vi "Read From I16 File.vi"(8 "start of read offset (bytes:0)":i32 caption="Start des Lese-Offset (Byte:0)", 9 "2D number of columns/1D count (all as 1D:-1)":i32=-1 caption="2D Spaltenanzahl/1D Anzahl (alle als 1D:-1)", 10 "2D number of rows":i32 caption="2D-Zeilenanzahl", 11 "file path (dialog if empty)":path caption="Dateipfad (Dialog, wenn leer)") -> (0 "mark after read (bytes)":i32 caption="Dateimarke nach Lesevorgang (Byte)", 1 "1D array":i16[](array[numeric]) caption="1D-Array", 2 "2D array":i16[][](array[numeric]) caption="2D-Array", 3 "new file path (Not A Path if cancelled)":path caption="Neuer Dateipfad (Kein Pfad, wenn abgebrochen)", 4 "EOF?":bool caption="Dateiende?")   [LabVIEW 2009]
doc: "Liest ein 2D- oder 1D-Daten-Array aus einer Bytestream-Datei mit vorzeichenbehafteten Word-Integern (I16) aus."
panel:
  in  "prompt":string="Zu lesende Datei wählen." caption="Eingabeaufforderung"
  in  "instructions":string="* Um die ganze Datei in ein 1D Array einzulesen, den 1D Zähler auf <0 (Standard) stellen ; Sie können die 2D Zeilenanzahl unverdrahtet lassen.\n* Zum Einlesen von N-Elementen in ein 1D Array, den 1D Zähler auf =N stellen und die 2D Zeilenanzahl verdrahtet lassen oder auf 0 stellen.\n* Zum Einlesen der ganzen Datei in ein 2D Array, die 2D Zeilenanzahl <auf 0 und die 2D Spaltenanzahl auf =N >0 stellen.  Das VI berechnet die Zeilenanzahl als integeren Teil der Dateigröße /N.\n* Zum Einlesen von M-Zeilen und N-Spalten in ein 2D Array, die 2D Zeilenanzahl auf =M und die 2D Spaltenanzahl auf =N stellen." caption="Anweisungen"
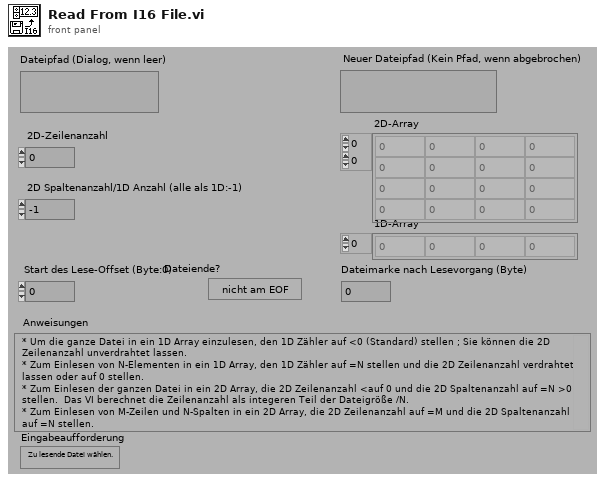
[diagram p1: front panel]
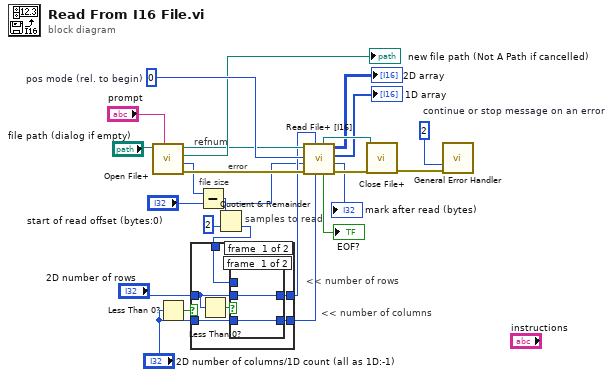
[diagram p0: block diagram]
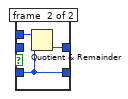
[diagram p2: hidden frame]
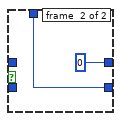
[diagram p3: hidden frame]
diagram:
  w21 = i16 0  # pos mode (rel. to begin)
  w22 = u16 2  # continue or stop message on an error
  # "samples to read"
  # "<< number of rows"
  # "<< number of columns"
  # "file size"
  # "error"
  # "refnum"
  n1 = call "Open File+.vi"("prompt"="prompt", "file path (\" \")"="file path (dialog if empty)") -> ("error out"=w23:errorcluster, "file size (bytes)"=w2:i32, "file path"=→"new file path (Not A Path if cancelled)":path, "refnum"=w12:refnum<file>)  [unwired: 6 in]
  n2 = Less Than 0?(x="2D number of columns/1D count (all as 1D:-1)") -> (x < 0?=w11:bool)
  n3 = Subtract(x=w2, y="start of read offset (bytes:0)") -> (x-y=w6:i32)
  n4 = Quotient & Remainder(x=w6, y=2) -> (floor(x/y)=w3:i32)  [unwired: 1 out]
  n5 = case shown="False" w11 {
    tunnel: [w29 0] -> w10
    tunnel: [w27 w36] -> w9
    tunnel: "2D number of columns/1D count (all as 1D:-1)" -> [w28 _]
    tunnel: "2D number of rows" -> [w25 _]
    tunnel: w3 -> [w26 w36]
    frame #0 {
      n6 = Less Than 0?(x=w25) -> (x < 0?=w30:bool)
      n7 = case shown="True" w30 {
        tunnel: [w31 w35] -> w29
        tunnel: w26 -> [_ w34]
        tunnel: w28 -> [w32 w33]
        tunnel: [w32 w33] -> w27
        tunnel: w25 -> [w31 _]
        frame #0 {
        }
        frame #1 {
          n8 = Quotient & Remainder(x=w34, y=w33) -> (floor(x/y)=w35:i32)  [unwired: 1 out]
        }
      }
    }
    frame #1 {
    }
  }
  n9 = call "Read File+ [I16].vi"("2D number of columns/1D count"=w9, "2D number of rows"=w10, "error in (no error)"=w23, "pos offset (bytes:0)"="start of read offset (bytes:0)", "pos mode (rel. to current:2)"=w21, "refnum"=w12) -> ("error out"=w20:errorcluster, "mark after read (bytes)"=→"mark after read (bytes)":i32, "1D data"=→"1D array":i16[], "2D data"=→"2D array":i16[][], "EOF?"=→"EOF?":bool, "dup refnum"=w16:refnum<file>)
  n10 = call "Close File+.vi"("error in (no error)"=w20, "refnum"=w16) -> ("error out"=w18:errorcluster)  [unwired: 3 in, 2 out]
  n11 = call <vilib>:"General Error Handler.vi"("type of dialog (OK msg:1)"=w22, "error in (no error)"=w18) -> ()  [unwired: 9 in, 5 out]
